vi "Read LogLevel.vi"(8 "error in (no error)":errorcluster, 11 "Log Sink in":refnum<class "Log Sink.lvclass">) -> (0 "error out":errorcluster, 2 "LogLevel":T1, 3 "Log Sink out":refnum<class "Log Sink.lvclass">)   [LabVIEW 2017, in "Composed Log.lvlib" / "Log Sink.lvclass"]
uses:
  Log Sink.lvclass
  Types/Log Level.ctl
  Log Sink.lvclass/Log Sink.ctl
  Composed Log.lvlib
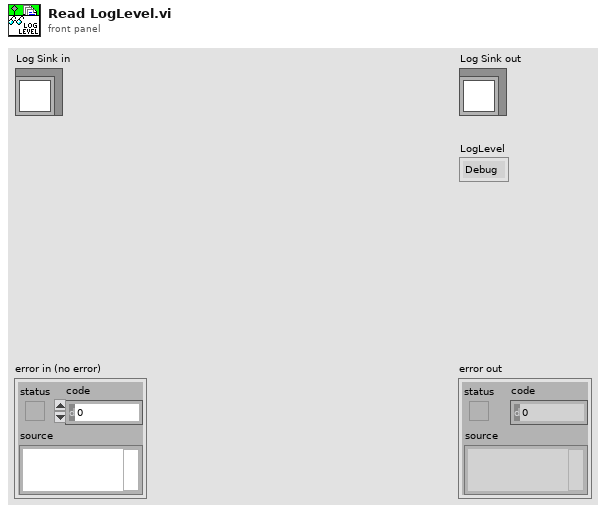
[diagram p1: front panel]
types:
  T1 = typedef "Composed Log.lvlib/Log Level.ctl" = enum16{"Debug", "Info", "Warning", "Error", "Critical"}
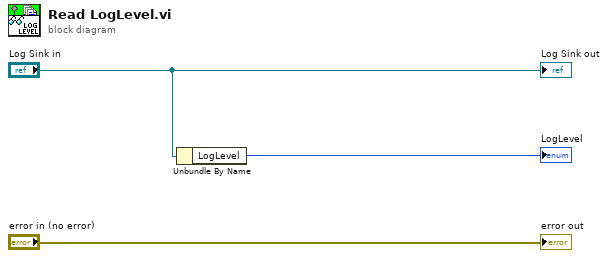
[diagram p0: block diagram]
diagram:
  n1 = Unbundle By Name("Log Sink in") -> ("LogLevel"=→"LogLevel":T1)
  "error out" <- "error in (no error)"
  "Log Sink out" <- "Log Sink in"
